vi "HapticSPM_write_test-bench.vi"() -> ()   [LabVIEW 2017]
uses:
  Program Files/National Instruments/LabVIEW 2019/user.lib/Haptic Prog Interface/Haptic Prog Interface.lvlib
  System.Windows.Forms
panel:
  in  "Function":string(combo)="0" caption="Combo Box"
  in  "Gain (mm/pm)":dbl=1.0 caption="Numeric" format="%.1g"
  in  "k":dbl=1.0 caption="Numeric" format="%.1g"
  in  "Setpoint":dbl=1e-10 caption="Numeric" format="%.0p"
  in  "Gain":dbl=1.0 caption="Numeric" format="%.1g"
  out "Value":dbl caption="Numeric" format="%#_2p"
  out "Click Number":dbl caption="Numeric" format="%#_1g"
  in  "Write Z":bool
  in  "Planing Toggle":bool
  in  "Planing Reset":bool
  in  "Save":bool
  in  "Stop":bool
  out "Frame Properties (m)":T1
  out "Surf Loc (m)":dbl
  out "Forces":T2 {"Fz (N)" format="%.1f"; "Fy (N)" format="%.1f"; "Fx (N)" format="%.1f"}
  out "Position (Reframed)":cluster{"x (m)":dbl, "y (m)":dbl, "z (mm)":dbl} {"z (mm)" format="%.0p"; "y (m)" format="%.1p"; "x (m)" format="%.1p"}
  out "Scan Window":refnum<k24>(container)
  # "Super Ultra Mega Haptic SPM Controller 3000"
  # "Scan Window"
  # "Signal"
  # "Force"
  # "Planing"
  # "Surface Scale"
  # "Z Write"
  # "Origin: X = Y = ;Width = Height = ;"
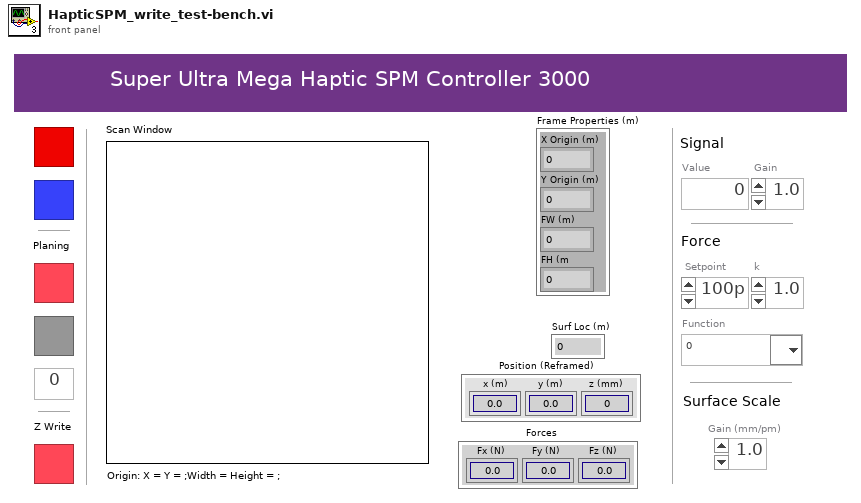
[diagram p1: front panel]
types:
  T1 = cluster{"X Origin (m)":dbl, "Y Origin (m)":dbl, "FW (m)":dbl, "FH (m":dbl}
  T2 = cluster{"Fx (N)":dbl, "Fy (N)":dbl, "Fz (N)":dbl}
  T3 = cluster{"kx (N/m)":dbl, "ky (N/m)":dbl, "kz (N/m)":dbl}
  T4 = cluster{"X Drag":bool, "Y Drag":bool, "Z Drag":bool}
  T5 = cluster{"x (mm)":dbl, "y (mm)":dbl, "z (mm)":dbl}
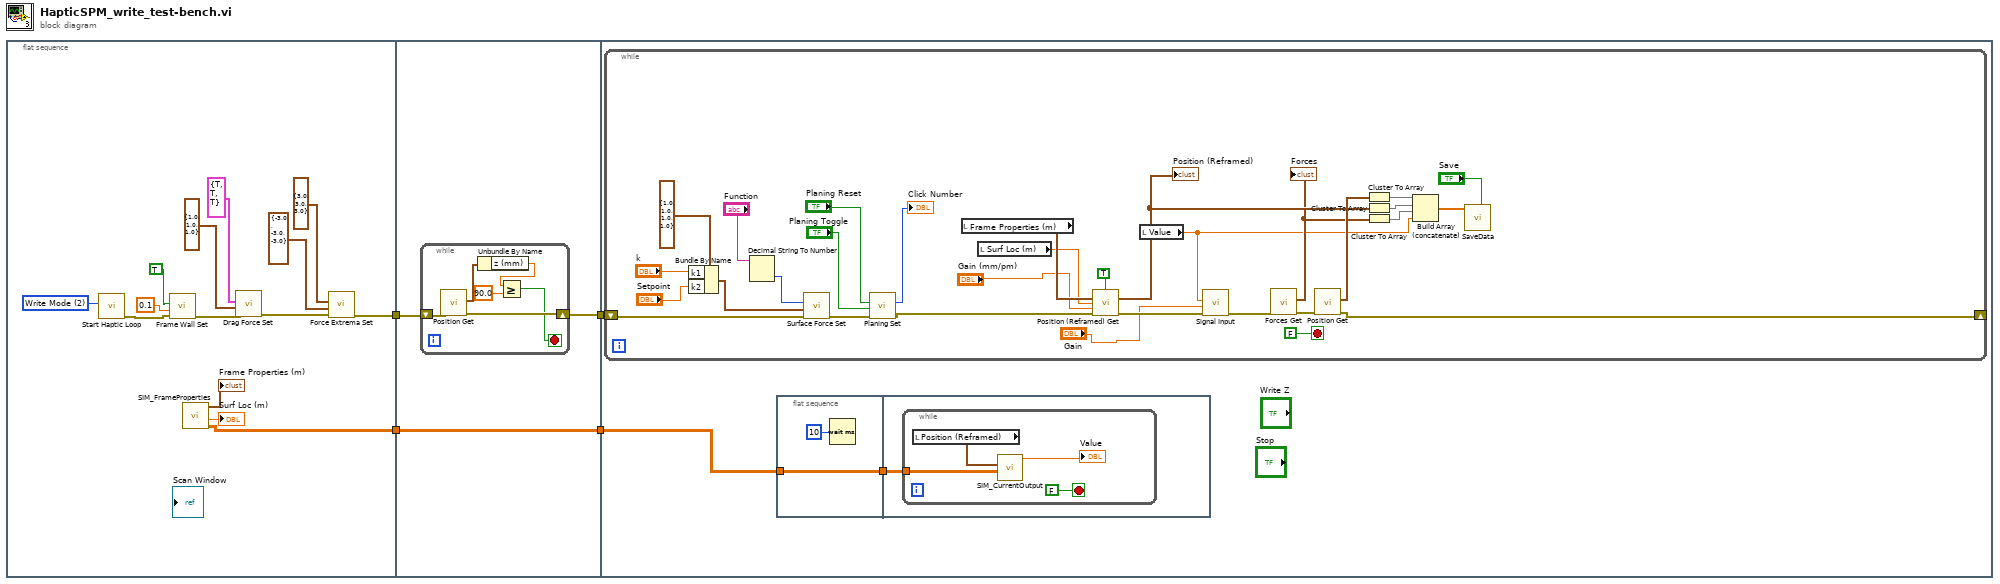
[diagram p0: block diagram]
diagram:
  n1 = flat-sequence {
    tunnel: [w16] -> w4
    tunnel: [w9] -> w2
    tunnel: w4 -> [w20]
    tunnel: [w19] -> w3
    tunnel: w2 -> [w21]
    tunnel: [w21] -> w1
    tunnel: w3 -> [w30]
    tunnel: w1 -> [w29]
    frame #0 {
      w18 = u16 2 items=["Custom Mode", "Read Mode", "Write Mode"] ("Mode Selection")
      n2 = call "Start Haptic Loop.vi"("Mode Selection"=w18) -> ("error out"=w6:errorcluster)  [unwired: 10 in]
      n3 = call "Frame Wall Set.vi"("error in (no error)"=w6, "Wall Stiffness (N/m)"=0.1 ("Wall Stiffness"), "Restrict to Frame"=TRUE) -> ("error out"=w5:errorcluster)  [unwired: 8 in]
      n4 = call "SIM_FrameProperties.vi"() -> ("data"=w9:dbl[][], "Surf Loc (m)"=→"Surf Loc (m)":dbl, "Center coordinates (m)"=→"Frame Properties (m)":cluster{"Xc":sgl, "Yc":sgl})  [unwired: 8 in, 1 out]
      n5 = call "Drag Force Set.vi"("error in (no error)"=w5, "Drag Coefficients (N/m)"=T3 {"kx (N/m)"=1.0, "ky (N/m)"=1.0, "kz (N/m)"=1.0} ("Drag Coefficients"), "Drag Force Toggles"=T4 {"X Drag"=TRUE, "Y Drag"=TRUE, "Z Drag"=TRUE}) -> ("error out"=w17:errorcluster)  [unwired: 8 in]
      n6 = call "Force Extrema Set.vi"("error in (no error)"=w17, "Minimum Force (N)"=T2 {"Fx (N)"=-3.0, "Fy (N)"=-3.0, "Fz (N)"=-3.0} ("Minimum Force"), "Maximum Force (N)"=T2 {"Fx (N)"=3.0, "Fy (N)"=3.0, "Fz (N)"=3.0} ("Maximum Force")) -> ("error out"=w16:errorcluster)  [unwired: 8 in]
    }
    frame #1 {
      n7 = while {
        shift-right: [w26] -> w19
        shift-left: w20 -> [w27]
        stop <- w22 stop-if-true
        n8 = call "Position Get.vi"("error in (no error)"=w27) -> ("error out"=w26:errorcluster, "Position"=w25:T5)  [unwired: 9 in]
        n9 = Unbundle By Name(w25) -> ("z (mm)"=w24:dbl)
        n10 = Greater Or Equal?(x=w24, y=90.0) -> (x >= y?=w22:bool)
      }
    }
    frame #2 {
      n11 = while {
        shift-right: [w59] -> _
        shift-left: w30 -> [w68]
        stop <- FALSE stop-if-true
        n12 = Bundle By Name(cluster=cluster{"k1":dbl, "k2":dbl, "k3":dbl, "k4":dbl} {"k1"=1.0, "k2"=1.0, "k3"=1.0, "k4"=1.0} ("Force Constants"), "k1"="k", "k2"="Setpoint") -> (w52:cluster{"k1":dbl, "k2":dbl, "k3":dbl, "k4":dbl})
        n13 = Decimal String To Number(string="Function") -> (number=w49:i32)  [unwired: 2 in, 1 out]
        n14 = call "Surface Force Set.vi"("error in (no error)"=w68, "Force Constants"=w52, "Force Settings"=w49) -> ("error out"=w67:errorcluster)  [unwired: 8 in]
        n15 = call "Planing Set.vi"("error in (no error)"=w67, "Planing"="Planing Toggle", "Reset"="Planing Reset") -> ("error out"=w55:errorcluster, "Number of Clicks"=→"Click Number":i8)  [unwired: 7 in]
        n16 = local read "Frame Properties (m)"() -> (w64:T1)
        n17 = local read "Surf Loc (m)"() -> (w63:dbl)
        n18 = call "Position (Reframed) Get.vi"("Z Rescaling"=TRUE, "Frame Properties (m)"=w64, "Surface Location (m)"=w63, "Scaling (mm per pm)"="Gain (mm/pm)", "error in (no error)"=w55) -> ("Reframed Position (m)"=w44:cluster{"x (m)":dbl, "y (m)":dbl, "z (m)":dbl}, "error out"=w61:errorcluster)  [unwired: 9 in]
        "Position (Reframed)" <- w44
        n19 = local read "Value"() -> (w40:dbl)
        n20 = call "Signal Input.vi"("error in (no error)"=w61, "Gain"="Gain", "Signal"=w40) -> ("error out"=w62:errorcluster)  [unwired: 8 in]
        n21 = call "Forces Get.vi"("error in (no error)"=w62) -> ("error out"=w60:errorcluster, "Force (N)"=w42:T2)  [unwired: 9 in]
        "Forces" <- w42
        n22 = call "Position Get.vi"("error in (no error)"=w60) -> ("error out"=w59:errorcluster, "Position"=w46:T5)  [unwired: 9 in]
        n23 = Cluster To Array(cluster=w46) -> (array=w45:dbl[])
        n24 = Cluster To Array(cluster=w44) -> (array=w43:dbl[])
        n25 = Cluster To Array(cluster=w42) -> (array=w41:dbl[])
        n26 = Build Array (concatenate)(w45, w43, w41, w40) -> (w39:dbl[])
        n27 = call "SaveData.vi"("Save"="Save", "Data"=w39) -> ()  [unwired: 10 in]
      }
      n28 = flat-sequence {
        tunnel: w29 -> [w32]
        tunnel: [w32] -> w28
        tunnel: w28 -> [w33]
        frame #0 {
          n29 = Wait (ms)(milliseconds to wait=u32 10) -> ()  [unwired: 1 out]
        }
        frame #1 {
          n30 = while {
            tunnel: w33 -> [w36]
            stop <- FALSE stop-if-true
            n31 = local read "Position (Reframed)"() -> (w35:cluster{"x (m)":dbl, "y (m)":dbl, "z (mm)":dbl})
            n32 = call "SIM_CurrentOutput.vi"("array"=w36, 10:w35) -> ("Current Out (A)"=→"Value":dbl)  [unwired: 8 in, 1 out]
          }
        }
      }
    }
  }
